vi "GetVoltage.vi"(4 "error in":errorcluster, 5 "connection ID":refnum<k5>) -> (0 "Voltage":string, 1 "error out":errorcluster, 2 "connection ID out":refnum<k5>, 3 "Answer":bool)   [LabVIEW 2013]
uses:
  <vilib>/regexp/Match Regular Expression.xnode
panel:
  out "output string":string
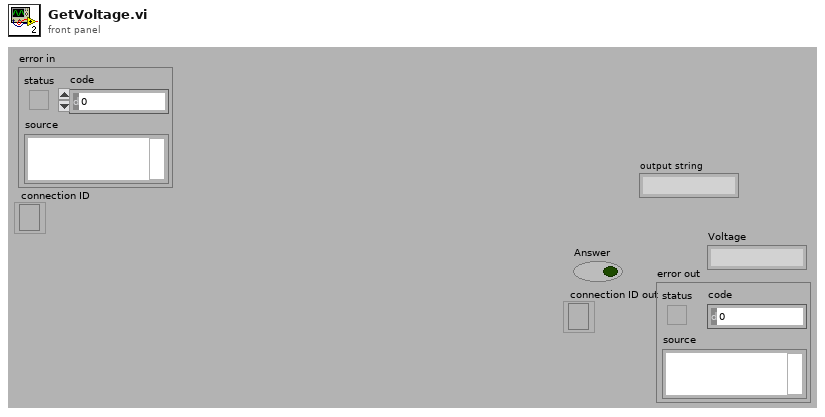
[diagram p1: front panel]
types:
  T1 = enum16{"Standard", "Buffered", "CRLF", "Immediate"}
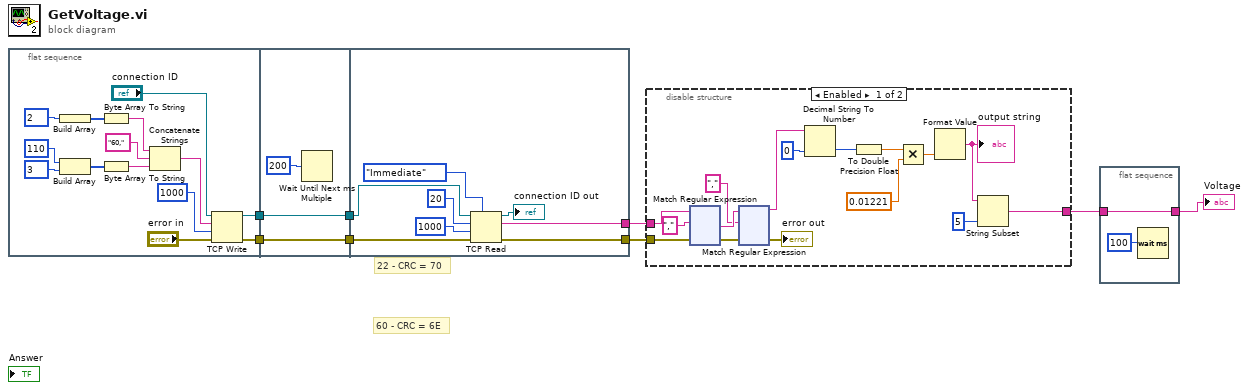
[diagram p0: block diagram]
diagram:
  # "60 - CRC = 6E"
  # "22 - CRC = 70"
  n1 = flat-sequence {
    tunnel: [w19] -> w7
    tunnel: [w18] -> w5
    tunnel: [w24] -> w8
    tunnel: w7 -> [w24]
    tunnel: [w23] -> w6
    tunnel: w5 -> [w23]
    tunnel: w8 -> [w29]
    tunnel: w6 -> [w28]
    tunnel: [w27] -> w4
    tunnel: [w26] -> w3
    frame #0 {
      n2 = Build Array(u8 2 ("y")) -> (w12:u8[])
      n3 = Build Array(u8 110 ("y"), u8 3 ("y")) -> (w16:u8[])
      n4 = Byte Array To String(unsigned byte array=w12) -> (string=w13:string)
      n5 = Byte Array To String(unsigned byte array=w16) -> (string=w17:string)
      n6 = Concatenate Strings(w13, "60," ("string"), w17) -> (w10:string)
      n7 = TCP Write(connection ID="connection ID", data in=w10, error in (no error)="error in", 9:1000 ("timeout ms (25000)")) -> (connection ID out=w19:refnum<k5>, error out=w18:errorcluster)  [unwired: 1 out]
    }
    frame #1 {
      n8 = Wait Until Next ms Multiple(millisecond multiple=u32 200) -> ()  [unwired: 1 out]
    }
    frame #2 {
      n9 = TCP Read(connection ID=w29, bytes to read=20, error in (no error)=w28, 7:T1."Immediate" ("mode (standard)"), 9:1000 ("timeout ms (25000)")) -> (connection ID out=→"connection ID out":refnum<k5>, data out=w27:string, error out=w26:errorcluster)
    }
  }
  n10 = disable-structure shown="Enabled" {
    disable-tunnel: w4 -> [w48 w278]
    disable-tunnel: w3 -> [w45 _]
    disable-tunnel: [w37 w278] -> w2
    frame Enabled {
      n11 = xnode "Match Regular Expression"("input string"=w48, "regular expression"=",", "error in"=w45) -> ("after match"=w47:string, "error out"=w44:errorcluster)  [unwired: 3 in, 3 out]
      n12 = xnode "Match Regular Expression"("input string"=w47, "regular expression"=",", "error in"=w44) -> ("before match"=w34:string, "error out"=→"error out":errorcluster)  [unwired: 3 in, 3 out]
      n13 = Decimal String To Number(string=w34, default (0L)=u32 0 ("default (0 I32)")) -> (number=w35:u32)  [unwired: 1 in, 1 out]
      n14 = To Double Precision Float(number=w35) -> (double precision float=w36:dbl)
      n15 = Multiply(x=w36, y=0.01221 ("default (0 I32)")) -> (x*y=w41:dbl)
      n16 = Format Value(value (0)=w41) -> (output string=w39:string)  [unwired: 2 in]
      "output string" <- w39
      n17 = String Subset(string=w39, length (rest)=5 ("length (rest)")) -> (substring=w37:string)  [unwired: 1 in]
    }
    frame Disabled {
    }
  }
  n18 = flat-sequence {
    tunnel: [w280] -> w1
    tunnel: w2 -> [w280]
    frame #0 {
      n19 = Wait (ms)(milliseconds to wait=u32 100) -> ()  [unwired: 1 out]
    }
  }
  "Voltage" <- w1
